vi "Get_Next_Sub_Collection.vi"(8 "error in (no error)":errorcluster caption="entrée d'erreur (pas d'erreur)", 11 "Firebase Benches en entrée":refnum<class "Firebase Benches_String.lvclass">) -> (0 "error out":errorcluster caption="sortie d'erreur", 3 "Firebase Benches en sortie":refnum<class "Firebase Benches_String.lvclass">)   [LabVIEW 2020, in "Library Instrument & Equipement.lvlib" / "Library FireBase.lvlib" / "Firebase Benches_String.lvclass"]
doc: "Return the documents present in the test collection for each DATA read with Get_Data\nPlease initialise the following values\n - Name BDD\n - Document of test sequence\n - API Key\n - Nb To Read"
uses:
  Firebase Benches_String.lvclass
  C:/Users/ngarcin/OneDrive - Altyor/Standard TB/Class/Firebase/Source/Firebase PCBA/Firebase Benches.lvclass
  C:/Users/ngarcin/OneDrive - Altyor/Standard TB/Class/Firebase/Source/Firebase Driver/Firebase Driver.lvclass
  Firebase Benches_String.lvclass/Firebase Benches_String.ctl
  JSON API/JSON Value/JSON Value.lvclass
  JSON API/JSON Value/Set from JSON string.vi
  Firebase Benches.lvclass
  JSON API/Variant JSON/Variant JSON.lvlib
  JSON API/Get Polymorphic/JSON GetSet.lvlib
  Firebase Driver/Firebase Driver.lvclass
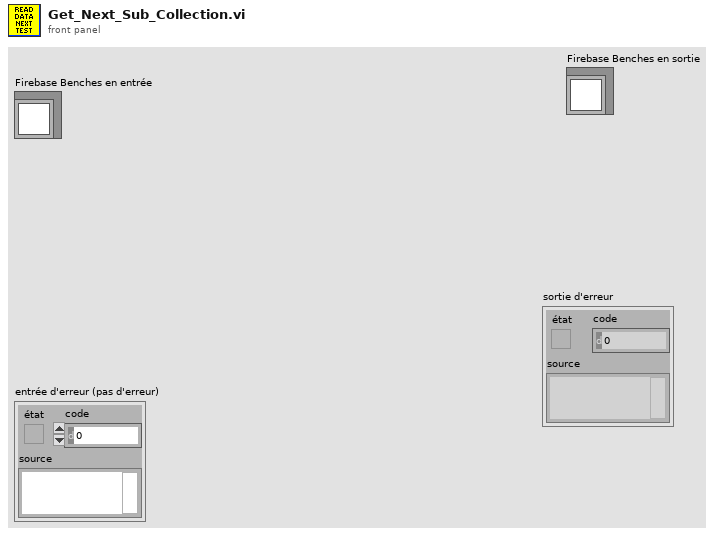
[diagram p1: front panel]
types:
  T1 = cluster{"name":string, "fields":cluster{"Result":cluster{"booleanValue":bool}, "Name":cluster{"stringValue":string}, "StartOfTest":cluster{"timestampValue":string}, "EndOfTest":cluster{"timestampValue":string}, "limit":cluster{"mapValue":cluster{"fields":cluster{"Lower":cluster{"stringValue":string}, "Upper":cluster{"stringValue":string}}}}, "Value":cluster{"stringValue":string}, "Type":cluster{"stringValue":string}, "MainTest":cluster{"stringValue":string}}}[][]
  T2 = cluster{"name":string, "fields":cluster{"Result":cluster{"booleanValue":bool}, "CreationDate":cluster{"timestampValue":string}, "Batch":cluster{"stringValue":string}, "SerialNumber":cluster{"stringValue":string}, "EndOfProduction":cluster{"timestampValue":string}, "FW_Version":cluster{"mapValue":cluster{"fields":cluster{"Bootloader":cluster{"mapValue":cluster{"fields":cluster{"File_Name":cluster{"stringValue":string}, "Version":cluster{"mapValue":cluster{"fields":cluster{"Major":cluster{"stringValue":string}, "Minor":cluster{"stringValue":string}}}}, "Checksum":cluster{"stringValue":string}}}}, "SoftDevice":cluster{"mapValue":cluster{"fields":cluster{"File_Name":cluster{"stringValue":string}, "Version":cluster{"mapValue":cluster{"fields":cluster{"Major":cluster{"stringValue":string}, "Minor":cluster{"stringValue":string}}}}, "Checksum":cluster{"stringValue":string}}}}, "DFU":cluster{"mapValue":cluster{"fields":cluster{"File_Name":cluster{"stringValue":string}, "Version":cluster{"mapValue":cluster{"fields":cluster{"Major":cluster{"stringValue":string}, "Minor":cluster{"stringValue":string}}}}, "Checksum":cluster{"stringValue":string}}}}}}}, "PartNumber":cluster{"stringValue":string}, "OrderNumber":cluster{"stringValue":string}, "Operator":cluster{"stringValue":string}}}[]
  T3 = cluster{"name":string, "fields":cluster{"Result":cluster{"booleanValue":bool}, "Name":cluster{"stringValue":string}, "StartOfTest":cluster{"timestampValue":string}, "EndOfTest":cluster{"timestampValue":string}, "limit":cluster{"mapValue":cluster{"fields":cluster{"Lower":cluster{"stringValue":string}, "Upper":cluster{"stringValue":string}}}}, "Value":cluster{"stringValue":string}, "Type":cluster{"stringValue":string}, "MainTest":cluster{"stringValue":string}}}[]
  T4 = cluster{"documents":cluster{"name":string, "fields":cluster{"Result":cluster{"booleanValue":bool}, "Name":cluster{"stringValue":string}, "StartOfTest":cluster{"timestampValue":string}, "EndOfTest":cluster{"timestampValue":string}, "limit":cluster{"mapValue":cluster{"fields":cluster{"Lower":cluster{"stringValue":string}, "Upper":cluster{"stringValue":string}}}}, "Value":cluster{"stringValue":string}, "Type":cluster{"stringValue":string}, "MainTest":cluster{"stringValue":string}}}[], "nextPageToken":string}
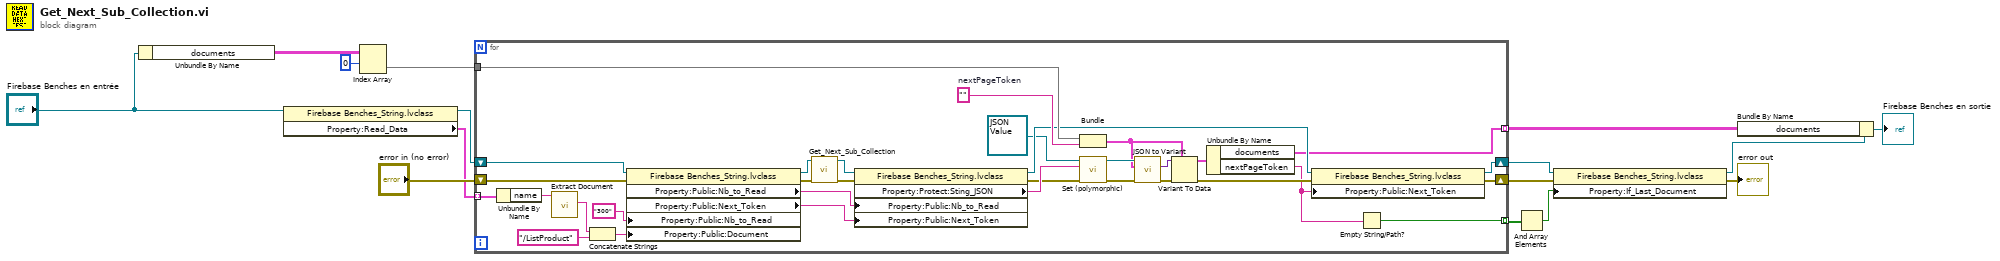
[diagram p0: block diagram]
diagram:
  n1 = Unbundle By Name("Firebase Benches en entrée") -> ("documents"=w14:T1)
  n2 = property class="Firebase Benches_String.lvclass"(reference="Firebase Benches en entrée") -> (reference out=w7:refnum<class "Firebase Benches_String.lvclass">, "Property:Read_Data"=w6:T2)  [unwired: 1 in, 1 out]
  n3 = Index Array(array=w14, index (row)=0 ("indice (ligne)")) -> (element=w13:T3)  [unwired: 1 in]
  n4 = for {
    tunnel: [w23] -> w15 mode=indexing
    shift-right: [w25] -> w4
    shift-left: w7 -> [w40]
    shift-right: [w27] -> w3
    shift-left: "error in (no error)" -> [w39]
    tunnel: w6 -> [w38] mode=indexing
    tunnel: w13 -> [w30]
    tunnel: [w16] -> w11 mode=indexing
    w42 = ""  # nextPageToken
    n5 = Unbundle By Name(w38) -> ("name"=w37:string)
    n6 = call "Extract Document.vi"("Name"=w37) -> ("Source"=w36:string)  [unwired: 9 in, 1 out]
    n7 = Concatenate Strings(w36, "/ListProduct" ("chaîne")) -> (w34:string)
    n8 = property class="Firebase Benches_String.lvclass"(reference=w40, error in=w39, "Property:Public:Nb_to_Read"="300" ("Nb_to_Read"), "Property:Public:Document"=w34) -> (reference out=w18:refnum<class "Firebase Benches_String.lvclass">, error out=w21:errorcluster, "Property:Public:Nb_to_Read"=w33:string, "Property:Public:Next_Token"=w31:string)
    n9 = call-parent "Get_Next_Sub_Collection.vi"("error in (no error)"=w21, "Firebase Benches en entrée"=w18) -> ("error out"=w20:errorcluster, "Firebase Benches en sortie"=w19:refnum<class "Firebase Benches_String.lvclass">)  [unwired: 8 in]
    n10 = property class="Firebase Benches_String.lvclass"(reference=w19, error in=w20, "Property:Public:Nb_to_Read"=w33, "Property:Public:Next_Token"=w31) -> (reference out=w26:refnum<class "Firebase Benches_String.lvclass">, error out=w29:errorcluster, "Property:Protect:Sting_JSON"=w44:string)
    n11 = Bundle("documents"=w30, "nextPageToken"=w42) -> (w41:T4)  [unwired: 1 in]
    n12 = call-poly "Set (polymorphic).vi"("error in (no error)"=w29, "JSON stream"=w44, "JSON Value in"=refnum<class "JSON Value.lvclass"> refnum) -> ("error out"=w45:errorcluster, "JSON Value out"=w47:refnum<class "JSON Value.lvclass">)  [unwired: 6 in, 1 out]
    n13 = call "JSON to Variant.vi"("error in (no error)"=w45, "Variant (Data Type)"=w41, "JSON Value"=w47) -> ("error out"=w46:errorcluster, "Variant out"=w22:variant)  [unwired: 7 in]
    n14 = Variant To Data(error in=w46, type=w41, Variant=w22) -> (data=w43:T4, error out=w28:errorcluster)
    n15 = Unbundle By Name(w43) -> ("documents"=w23:T3, "nextPageToken"=w17:string)
    n16 = property class="Firebase Benches_String.lvclass"(reference=w26, error in=w28, "Property:Public:Next_Token"=w17) -> (reference out=w25:refnum<class "Firebase Benches_String.lvclass">, error out=w27:errorcluster)
    n17 = Empty String/Path?(string/path=w17) -> (empty?=w16:bool)
  }
  n18 = And Array Elements(Boolean array=w11) -> (logical AND=w5:bool)
  n19 = property class="Firebase Benches_String.lvclass"(reference=w4, error in=w3, "Property:If_Last_Document"=w5) -> (reference out=w2:refnum<class "Firebase Benches_String.lvclass">, error out=→"error out":errorcluster)
  n20 = Bundle By Name(cluster=w2, "documents"=w15) -> (→"Firebase Benches en sortie":refnum<class "Firebase Benches_String.lvclass">)
